vi "Cyclic.vi"(7 "Reinit":bool, 8 "error in (no error)":errorcluster, 10 "X":i64, 11 "Stats_I64_CIF_U in":refnum<class "Stats_I64_CIF_U.lvclass">) -> (0 "error out":errorcluster, 3 "Stats_I64_CIF_U out":refnum<class "Stats_I64_CIF_U.lvclass">)   [LabVIEW 2021, in "Stats_CIF_U.lvlib" / "Stats_I64_CIF_U.lvclass"]
doc: "Load a new data value into the statistics class. The new value will be calculated by subracting the new X value from the last value added to the class. This VI is useful for cyclic timing where timestamps are provided as input X."
uses:
  Stats_I64_CIF_U.lvclass
  Stats_I64_CIF_U.lvclass/Stats_I64_CIF_U.ctl
  dfabcf33-0dbc-4041-80a5-3dc0c86d2989.vi
  dfabcf33-0dbc-4041-80a5-3dc0c86d2989.vi/9eb60a9a-770f-4d2d-8b3f-8465c267ecc9.vi
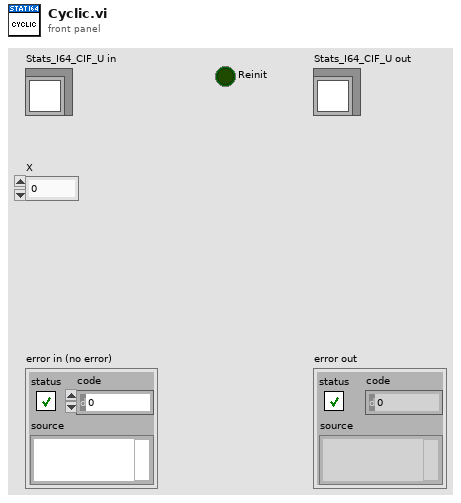
[diagram p1: front panel]
types:
  T1 = typedef "Stats_CIF_U.lvlib/I64 Stat Data.ctl" = cluster{"Last Value":i64, "Max":i64, "Min":i64, "Common ":T2}
  T2 = typedef "Stats_CIF_U.lvlib/Common Stat Data.ctl" = cluster{"Iteration":u32, "Max History":i32, "Average":dbl, "Init":bool}
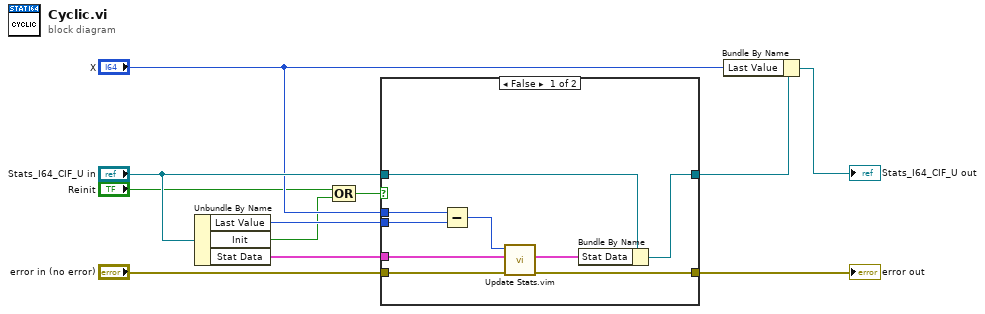
[diagram p0: block diagram]
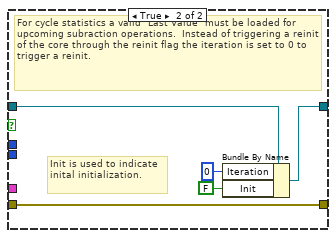
[diagram p2: hidden frame]
diagram:
  n1 = Unbundle By Name("Stats_I64_CIF_U in") -> ("Last Value"=w8:i64, "Init"=w1:bool, "Stat Data"=w7:T1)
  n2 = Compound Arithmetic op=OR("Reinit", w1) -> (w2:bool)
  n3 = case shown="False" w2 {
    tunnel: "error in (no error)" -> [w20 w25]
    tunnel: [w18 w25] -> w10
    tunnel: "Stats_I64_CIF_U in" -> [w17 w24]
    tunnel: w8 -> [w16 _]
    tunnel: w7 -> [w15 _]
    tunnel: "X" -> [w14 _]
    tunnel: [w13 w23] -> w5
    frame False {
      n4 = Subtract(x=w14, y=w16) -> (x-y=w12:i64)
      n5 = call "Update Stats.vim"("error in"=w20, "Stat Data In"=w15, "New Value"=w12) -> ("error out"=w18:errorcluster, "Stat Data Out"=w19:T1)  [unwired: 7 in]
      n6 = Bundle By Name(cluster=w17, "Stat Data"=w19) -> (w13:refnum<class "Stats_I64_CIF_U.lvclass">)
    }
    frame True {
      # "Init is used to indicate inital initialization."
      # "For cycle statistics a valid \"Last Value\" must be loaded for upcoming subraction operations.  Instead of triggering a reinit of the core through the reinit flag the iteration is set to 0 to trigger a reinit."
      n7 = Bundle By Name(cluster=w24, "Iteration"=u32 0 ("Stat Data.Common .Iteration"), "Init"=FALSE ("Stat Data.Common .Init")) -> (w23:refnum<class "Stats_I64_CIF_U.lvclass">)
    }
  }
  "error out" <- w10
  n8 = Bundle By Name(cluster=w5, "Last Value"="X") -> (→"Stats_I64_CIF_U out":refnum<class "Stats_I64_CIF_U.lvclass">)
